vi "Capteur avec Keller - Version demo.vi"(7 "XY Graph Ref In":refnum<vi>, 9 "Length":i32=250, 11 "Online":bool) -> (3 "Value":sgl(graph))   [LabVIEW 2013]
uses:
  <vilib>/Utility/config.llb/Read Key (String).vi
  <vilib>/Utility/config.llb/Read Key (U32).vi
  SubVI/K_S30c_VISA/K_S30c_VISA.lvlib
  <vilib>/Utility/config.llb/NI_LVConfig.lvlib
panel:
  out "Pressure":cluster{"Y":dbl[], "Y":dbl[]}[](graph)
  in  "Address":u8=250
  in  "Channel":enum16{"CH0", "P1", "P2", "T", "TOB1", "TOB2"}(ring)=enum."P1"
  out "error":errorcluster
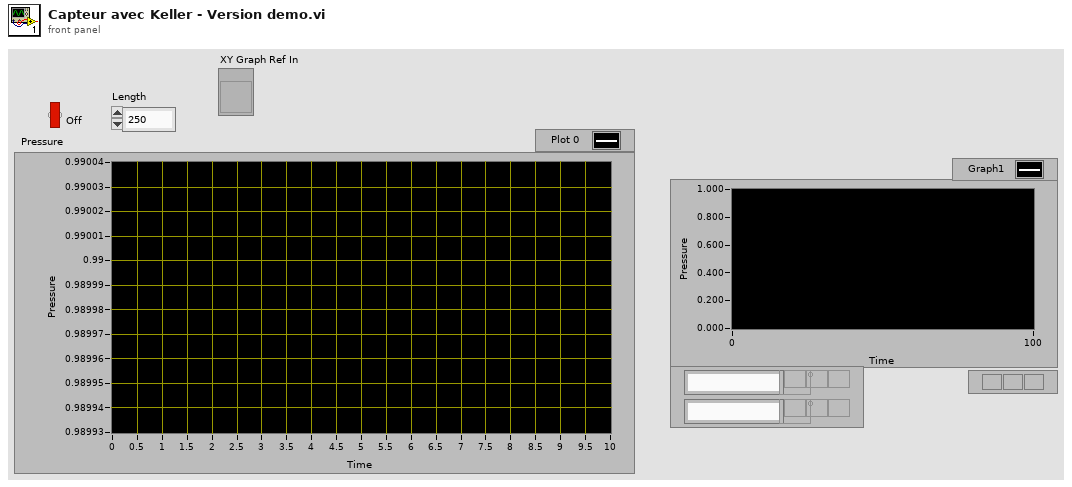
[diagram p1: front panel]
types:
  T1 = typedef "NI_LVConfig.lvlib/Config Data RefNum.ctl" = refnum<k1>
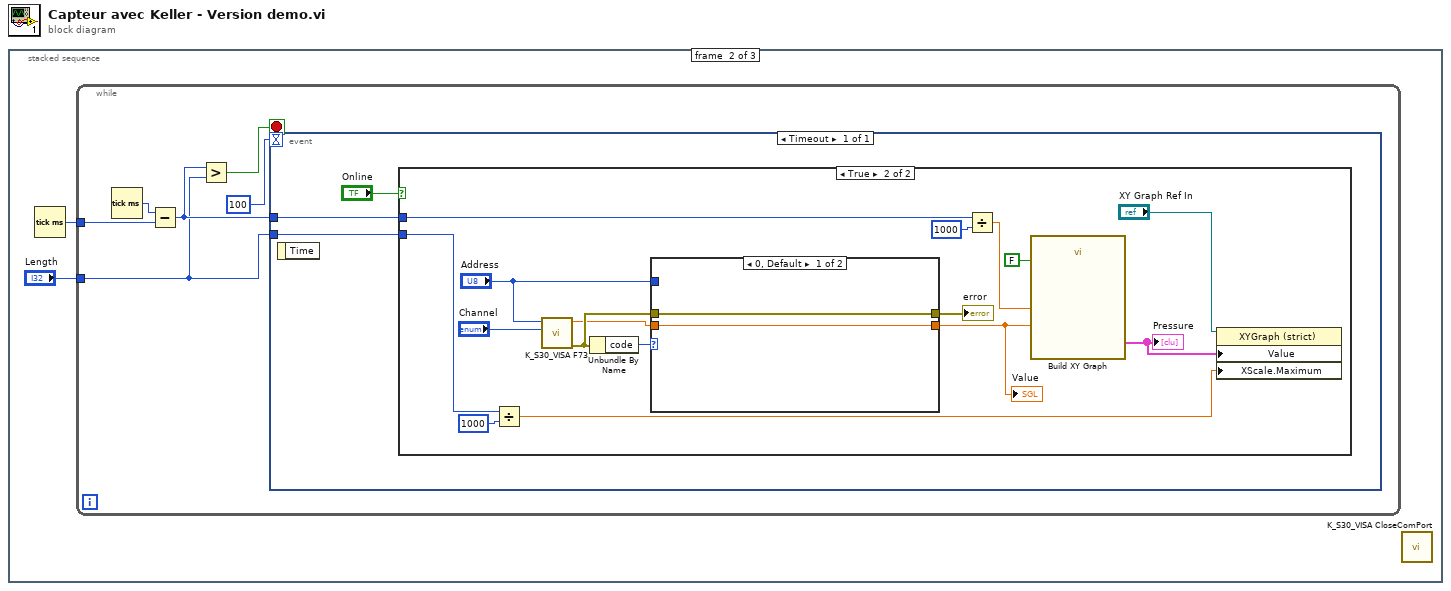
[diagram p0: block diagram]
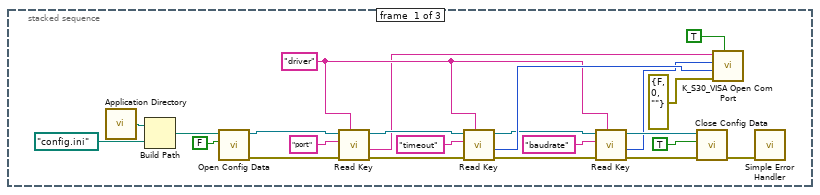
[diagram p2: hidden frame]
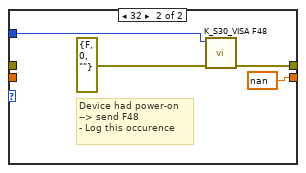
[diagram p4: hidden frame]
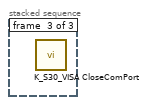
[diagram p5: hidden frame]
diagram:
  n1 = stacked-sequence {
    frame #0 {
      w4 = "driver" ("section")
      n2 = call <vilib>:"Application Directory.vi"() -> ("Application Directory"=w13:path)
      n3 = Build Path(base path=w13, name or relative path=path "config.ini" ("default name")) -> (appended path=w17:path)
      n4 = call <vilib>:"Open Config Data.vi"("create file if necessary (T)"=FALSE ("create file if necessary? (T)"), "configuration file path"=w17) -> ("error out"=w16:errorcluster, "refnum"=w14:T1)  [unwired: 7 in, 1 out]
      n5 = call-poly <vilib>:"Read Key.vi"("section"=w4, "error in (no error)"=w16, "key"="port", "refnum"=w14) -> ("error out"=w11:errorcluster, "value"=w1:string, "refnum out"=w12:T1)  [unwired: 4 in, 1 out]
      n6 = call-poly <vilib>:"Read Key.vi"("section"=w4, "error in (no error)"=w11, "key"="timeout", "refnum"=w12) -> ("error out"=w5:errorcluster, "value"=w9:u32, "refnum out"=w8:T1)  [unwired: 4 in, 1 out]
      n7 = call-poly <vilib>:"Read Key.vi"("section"=w4, "error in (no error)"=w5, "key"="baudrate", "refnum"=w8) -> ("error out"=w6:errorcluster, "value"=w3:u32, "refnum out"=w7:T1)  [unwired: 4 in, 1 out]
      n8 = call <vilib>:"Close Config Data.vi"("error in (no error)"=w6, "write file if changed (T)"=TRUE ("write configuration file? (T)"), "refnum"=w7) -> ("error out"=w19:errorcluster)  [unwired: 8 out]
      n9 = call "K_S30_VISA Open Com Port.vi"("RS-converter:\necho"=TRUE ("RS-converter: echo"), "error in (no error)"=errorcluster {"status"=FALSE, "code"=0, "source"=""}, "timeout"=w9, "Baudrate"=w3, "VISA resource name"=w1) -> ()  [unwired: 3 in, 2 out]
      n10 = call <vilib>:"Simple Error Handler.vi"("error in (no error)"=w19) -> ()  [unwired: 1 in, 8 out]
    }
    frame #1 {
      n11 = Tick Count (ms)() -> (millisecond timer value=w24:u32)
      n12 = while {
        tunnel: "Length" -> [w26]
        tunnel: w24 -> [w29]
        stop <- w28 stop-if-true
        n13 = Tick Count (ms)() -> (millisecond timer value=w30:u32)
        n14 = Subtract(x=w30, y=w29) -> (x-y=w27:u32)
        n15 = Greater?(x=w27, y=w26) -> (0:w28:bool)
        n16 = event shown="[0] Timeout" {
          selector: _ -> [_]
          dyn-events: _ -> [_]
          timeout: 100 -> [_]
          tunnel: w27 -> [w33]
          tunnel: w26 -> [w32]
          event Timeout {
            n17 = event-data() -> ()  [unwired: 1 in, 1 out]
            n18 = case shown="True" "Online" {
              tunnel: w33 -> [_ w40]
              tunnel: w32 -> [_ w37]
              frame False {
              }
              frame True {
                n19 = Divide(x=w37, y=1000) -> (x/y=w38:dbl)
                n20 = call "K_S30_VISA F73.vi"("Channel"="Channel", "Address"="Address") -> ("error out"=w47:errorcluster, "Value"=w46:sgl)  [unwired: 3 in, 1 out]
                n21 = Unbundle By Name(w47) -> ("code"=w49:i32)
                n22 = case shown="0, Default" w49 {
                  tunnel: "Address" -> [_ w55]
                  tunnel: w47 -> [w51 _]
                  tunnel: w46 -> [w52 _]
                  tunnel: [w52 sgl nan] -> w35
                  tunnel: [w51 w53] -> w45
                  frame 0, Default {
                  }
                  frame 32 {
                    # "Device had power-on\n--> send F48\n- Log this occurence"
                    n23 = call "K_S30_VISA F48.vi"("error in"=errorcluster {"status"=FALSE, "code"=0, "source"=""}, "Address"=w55) -> ("error out"=w53:errorcluster)  [unwired: 3 in, 2 out]
                  }
                }
                "error" <- w45
                "Value" <- w35
                n24 = Divide(x=w40, y=1000) -> (x/y=w41:dbl)
                n25 = call "Build XY Graph"("Reset"=FALSE, "Y Input"=w35, "X Input"=w41) -> ("XY Graph"=w42:cluster{"Y":dbl[], "Y":dbl[]}[])  [unwired: 2 in, 6 out]
                "Pressure" <- w42
                n26 = property class="XYGraph (strict)"(reference="XY Graph Ref In", "Value"=w42, "XScale.Maximum"=w38) -> ()  [unwired: 1 in, 2 out]
              }
            }
          }
        }
      }
      n27 = call "K_S30_VISA CloseComPort.vi"() -> ()  [unwired: 7 in, 1 out]
    }
    frame #2 {
      n28 = call "K_S30_VISA CloseComPort.vi"() -> ()  [unwired: 7 in, 1 out]
    }
  }
